vi "Close XL Application.vi"(8 "error in":errorcluster, 11 "Excel._Application":refnum<k7>) -> (0 "error out":errorcluster)   [LabVIEW 2017]
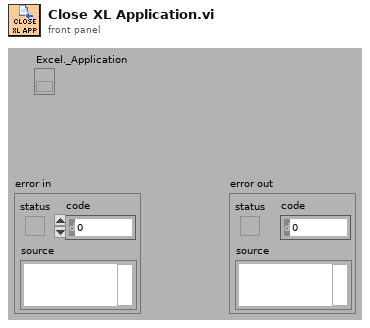
[diagram p1: front panel]
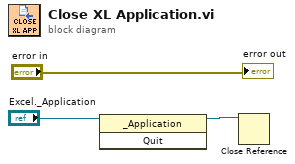
[diagram p0: block diagram]
diagram:
  n1 = invoke class="_Application" method="Quit"(reference="Excel._Application") -> (reference out=w3:refnum<k7>)  [unwired: 2 in, 2 out]
  n2 = Close Reference(reference=w3) -> ()  [unwired: 1 in, 1 out]
  "error out" <- "error in"
